vi "PS Analyze Power Measurements.vi"(0 "Voltage Waveform In":waveform(dbl), 5 "Current Waveform In":waveform(dbl), 11 "error in (no error)":errorcluster) -> (4 "Power Measurements":T1 {"Average Power (W)" format="%#.2p"; "Max Power(W)" format="%#.2p"; "Max Current Level(A)" format="%#.2p"; "Max Voltage Level(V)" format="%#.2p"}, 15 "error out":errorcluster)   [LabVIEW 2021, in "DAQ_Power Supply Source and Measure.lvlib"]
doc: "Analyzes the power voltage and current waveform data to derive required power measurments"
uses:
  DAQ_Power Supply Source and Measure.lvlib
  Typedefs/Power Measurements.ctl
  <vilib>/Analysis/baseanly.llb/Mean (DBL).vi
  <vilib>/Analysis/NI_AALBase.lvlib
panel:
  # "Inputs"
  # "Outputs"
  # "Overview:\nThis VI does post processing on obtained voltage and current waveform from power supply measurements to give the required Power Measurements output\n\nInstructions:\n1. Input the captured voltage and current waveform to the input controls\n2. Observe the analyzed power measurements output"
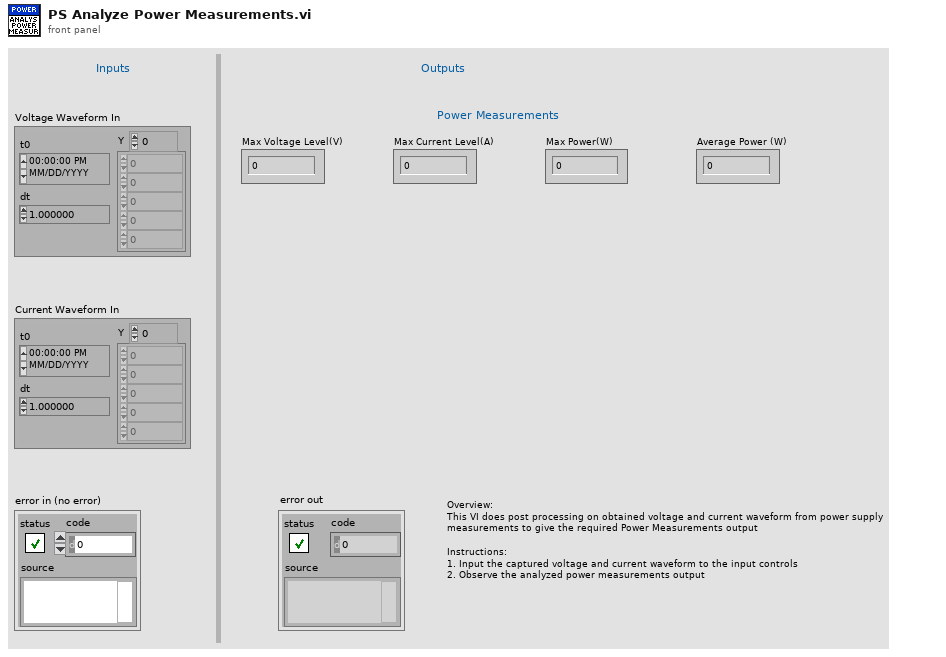
[diagram p1: front panel]
types:
  T1 = typedef "DAQ_Power Supply Source and Measure.lvlib/Power Measurements.ctl" = cluster{"Max Voltage Level(V)":dbl, "Max Current Level(A)":dbl, "Max Power(W)":dbl, "Average Power (W)":dbl}
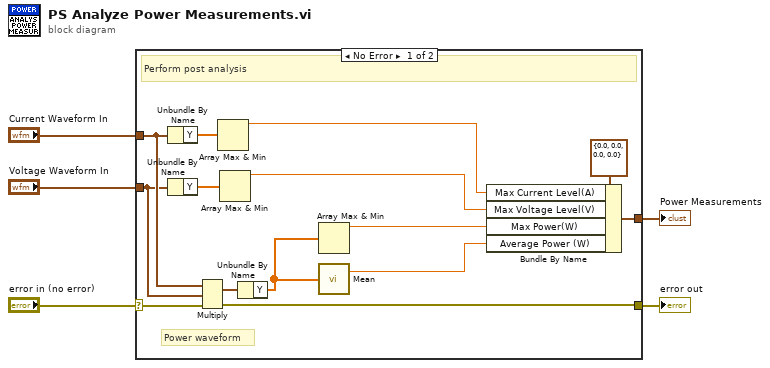
[diagram p0: block diagram]
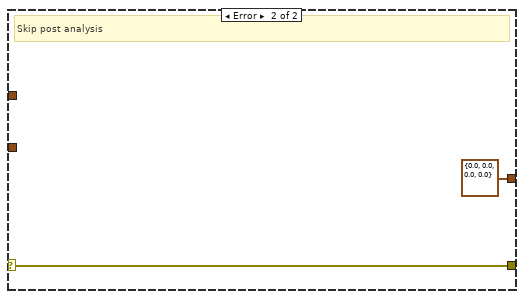
[diagram p2: hidden frame]
diagram:
  n1 = case shown="No Error" "error in (no error)" {
    selector: "error in (no error)" -> [w13 w21]
    tunnel: [w19 T1 {"Max Voltage Level(V)"=0.0, "Max Current Level(A)"=0.0, "Max Power(W)"=0.0, "Average Power (W)"=0.0} ("Power Measurements")] -> w5
    tunnel: "Current Waveform In" -> [w15 _]
    tunnel: [w12 w21] -> w2
    tunnel: "Voltage Waveform In" -> [w14 _]
    frame No Error {
      # "Power waveform"
      # "Perform post analysis"
      n2 = Unbundle By Name(w15) -> ("Y"=w8:dbl[])
      n3 = Unbundle By Name(w14) -> ("Y"=w7:dbl[])
      n4 = Multiply(1:w14, 2:w15, 4:w13) -> (0:w11:waveform(dbl), 3:w12:errorcluster)
      n5 = Array Max & Min(array=w8) -> (max value=w17:dbl)  [unwired: 3 out]
      n6 = Array Max & Min(array=w7) -> (max value=w16:dbl)  [unwired: 3 out]
      n7 = Unbundle By Name(w11) -> ("Y"=w6:dbl[])
      n8 = Array Max & Min(array=w6) -> (max value=w10:dbl)  [unwired: 3 out]
      n9 = call-poly <vilib>:"Mean.vi"("X"=w6) -> ("mean"=w9:dbl)  [unwired: 1 out]
      n10 = Bundle By Name(cluster=T1 {"Max Voltage Level(V)"=0.0, "Max Current Level(A)"=0.0, "Max Power(W)"=0.0, "Average Power (W)"=0.0} ("Power Measurements"), "Max Current Level(A)"=w17, "Max Voltage Level(V)"=w16, "Max Power(W)"=w10, "Average Power (W)"=w9) -> (w19:T1)
    }
    frame Error {
      # "Skip post analysis"
    }
  }
  "error out" <- w2
  "Power Measurements" <- w5
